vi "APS set point table3.vi"(7 "Point":T1, 8 "error in (no error)":errorcluster caption="错误输入（无错误）", 9 "Index":i32, 10 "Axis_ID_Array":i32, 11 "Dimension":i32) -> (0 "error out":errorcluster caption="错误输出", 2 "Axis_ID_Array out":i32, 3 "function return":i32, 5 "Point out":T1)   [LabVIEW 2011, in "APS168.lvlib"]
doc: "I32 FNTYPE APS_set_point_table3( I32 Dimension, I32 *Axis_ID_Array, I32 Index, POINT_DATA3 *Point );"
uses:
  APS168.lvlib
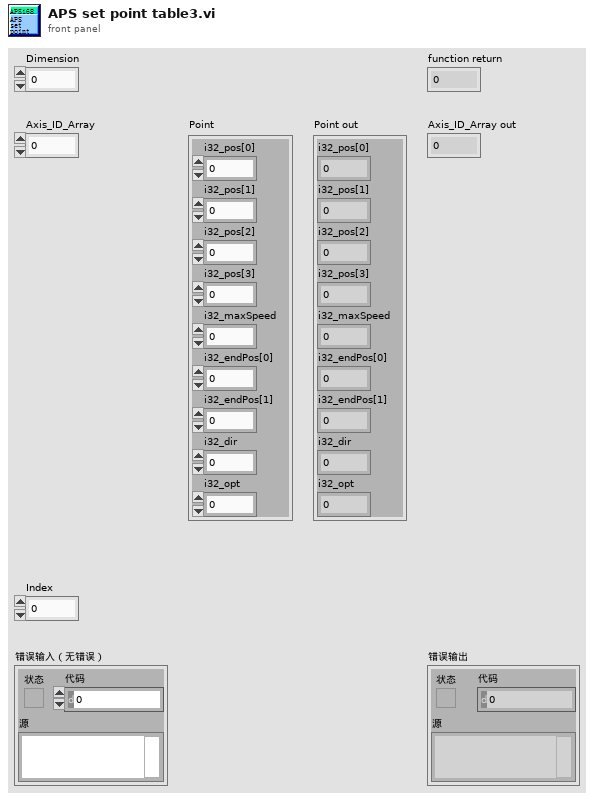
[diagram p1: front panel]
types:
  T1 = cluster{"i32_pos[0]":i32, "i32_pos[1]":i32, "i32_pos[2]":i32, "i32_pos[3]":i32, "i32_maxSpeed":i32, "i32_endPos[0]":i32, "i32_endPos[1]":i32, "i32_dir":i32, "i32_opt":i32}
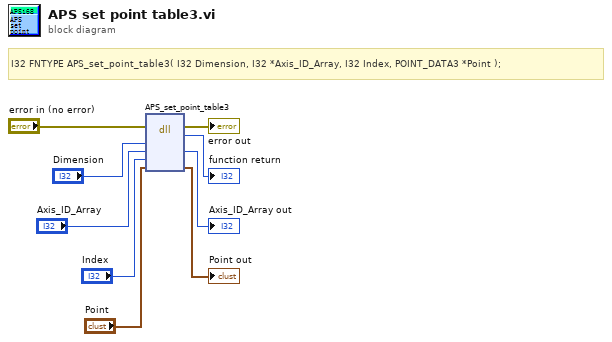
[diagram p0: block diagram]
diagram:
  # "I32 FNTYPE APS_set_point_table3( I32 Dimension, I32 *Axis_ID_Array, I32 Index, POINT_DATA3 *Point );"
  n1 = dll-call lib="PTH1Labs E软件ADLINK 204CAPS_1_7_1_LIB line 连续运动204APS168.*" fn="APS_set_point_table3"(error in="error in (no error)", "Dimension"="Dimension", "Axis_ID_Array"="Axis_ID_Array", "Index"="Index", "Point"="Point") -> (error out=→"error out":errorcluster, →"function return":i32, "Axis_ID_Array"=→"Axis_ID_Array out":i32, "Point"=→"Point out":T1)  [unwired: 4 in, 1 out]
